vi "terminate.vi"(8 "error in (no error)":errorcluster, 11 "DL090602SutterMP285Stage in":refnum<class "StageDL090602SutterMP285.lvclass">) -> (0 "error out":errorcluster, 3 "DL090602SutterMP285Stage out":refnum<class "StageDL090602SutterMP285.lvclass">)   [LabVIEW 2010, in "StageDL090602SutterMP285.lvclass"]
doc: "The dynamic dispatch version of this VI terminates the plug-in object by releasing all of its resources."
uses:
  StageDL090602SutterMP285.lvclass
  StageDL090602SutterMP285.lvclass/StageDL090602SutterMP285.ctl
  StageDL090409Scaffold/StageDL090409Scaffold/StageDL090409Scaffold.lvclass
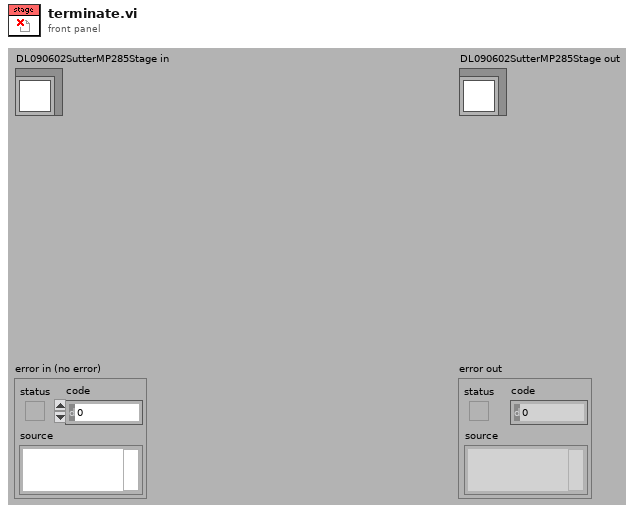
[diagram p1: front panel]
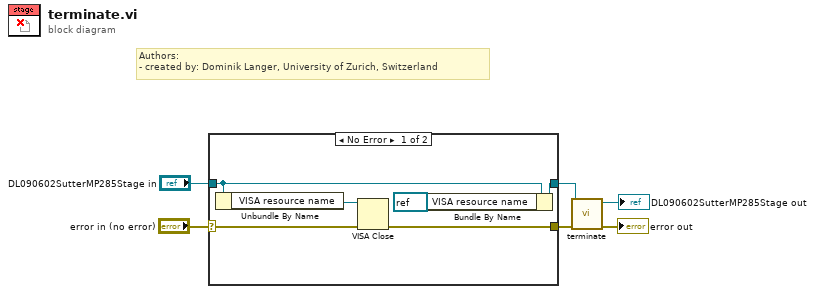
[diagram p0: block diagram]
diagram:
  # "Authors: \n- created by: Dominik Langer, University of Zurich, Switzerland"
  n1 = case shown="No Error" "error in (no error)" {
    selector: "error in (no error)" -> [w11 w13]
    tunnel: "DL090602SutterMP285Stage in" -> [w9 w14]
    tunnel: [w8 w14] -> w2
    tunnel: [w12 w13] -> w1
    frame No Error {
      n2 = Unbundle By Name(w9) -> ("VISA resource name"=w10:refnum<visa-resource-name>)
      n3 = VISA Close(VISA resource name=w10, error in (no error)=w11) -> (error out=w12:errorcluster)
      n4 = Bundle By Name(cluster=w9, "VISA resource name"=refnum<visa-resource-name> refnum) -> (w8:refnum<class "StageDL090602SutterMP285.lvclass">)
    }
    frame Error {
    }
  }
  n5 = call-parent "terminate.vi"("error in (no error)"=w1, "GenericPlugin in"=w2) -> ("error out"=→"error out":errorcluster, "GenericPlugin out"=→"DL090602SutterMP285Stage out":refnum<class "StageDL090602SutterMP285.lvclass">)  [unwired: 8 out]
